vi "AbsWindToRelWind.vi"(9 "Boat Speed":dbl, 10 "Absolute Wind Direction":dbl, 11 "Absolute Wind Speed":dbl) -> (1 "Relative Wind Direction":dbl, 2 "Relative Wind Speed":dbl)   [LabVIEW 2013]
doc: "In the pool, we can set the absolute wind direction and speed using the fans, but the little boat does not currently have a functional wind sensor, so we must calculate relative wind.\n\nThis VI calculates relative wind using the given absolute wind direction and speed as well as the measured boat speed.\n\n-Elizabeth Mahon, 4/12/2014"
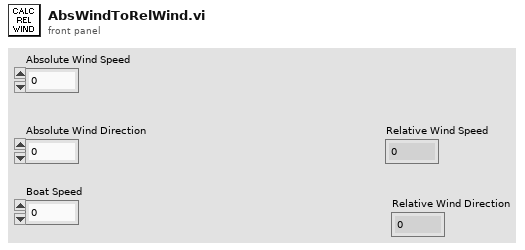
[diagram p1: front panel]
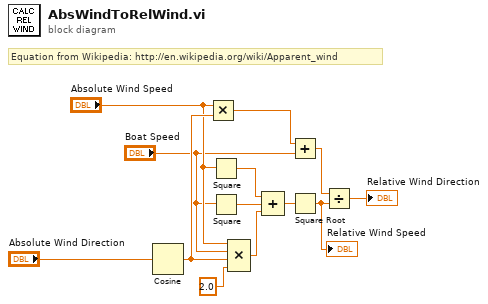
[diagram p0: block diagram]
diagram:
  # "Equation from Wikipedia: http://en.wikipedia.org/wiki/Apparent_wind"
  n1 = Cosine(x="Absolute Wind Direction") -> (cos(x)=w4:dbl)
  n2 = Multiply(x="Absolute Wind Speed", y=w4) -> (x*y=w5:dbl)
  n3 = Square(x="Absolute Wind Speed") -> (x^2=w12:dbl)
  n4 = Square(x="Boat Speed") -> (x^2=w11:dbl)
  n5 = Compound Arithmetic op=MULTIPLY("Absolute Wind Speed", "Boat Speed", w4, 2.0 ("value")) -> (w9:dbl)
  n6 = Compound Arithmetic op=ADD(w12, w11, w9) -> (w13:dbl)
  n7 = Add(x=w5, y="Boat Speed") -> (x+y=w6:dbl)
  n8 = Square Root(x=w13) -> (sqrt(x)=w7:dbl)
  "Relative Wind Speed" <- w7
  n9 = Divide(x=w6, y=w7) -> (x/y=→"Relative Wind Direction":dbl)
